vi "GraphXYto2DArrayIndexes.vi"(8 "error in (no error)":errorcluster, 10 "XY":cluster{"X":dbl, "Y":dbl}, 11 "IntensityGraph in":refnum<vi>) -> (0 "error out":errorcluster, 1 "Y Index":i32, 2 "X Index":i32, 3 "reference out":refnum<vi>)   [LabVIEW 2023]
doc: "This VI translates axis position Coord on the graph to it's nearest X and Y pixel index."
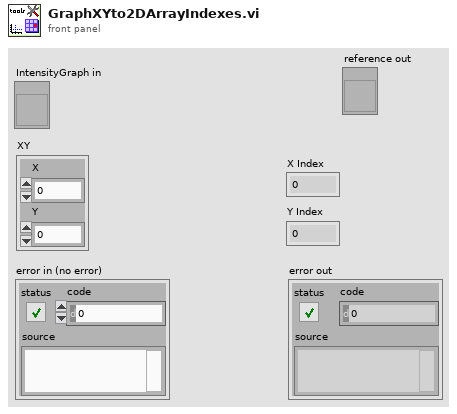
[diagram p1: front panel]
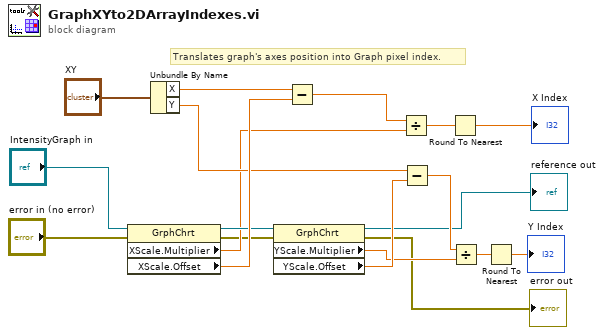
[diagram p0: block diagram]
diagram:
  # "Translates graph's axes position into Graph pixel index."
  n1 = property on="Property Node" class="GrphChrt"(reference="IntensityGraph in", error in="error in (no error)") -> (reference out=w10:refnum<vi>, error out=w4:errorcluster, "XScale.Multiplier"=w8:dbl, "XScale.Offset"=w15:dbl)
  n2 = Unbundle By Name("XY") -> ("X"=w14:dbl, "Y"=w12:dbl)
  n3 = property on="Property Node" class="GrphChrt"(reference=w10, error in=w4) -> (reference out=→"reference out":refnum<vi>, error out=→"error out":errorcluster, "YScale.Multiplier"=w11:dbl, "YScale.Offset"=w13:dbl)
  n4 = Subtract(x=w14, y=w15) -> (x-y=w7:dbl)
  n5 = Divide(x=w7, y=w8) -> (x/y=w16:dbl)
  n6 = Subtract(x=w12, y=w13) -> (x-y=w9:dbl)
  n7 = Round To Nearest(number=w16) -> (nearest integer value=→"X Index":dbl)
  n8 = Divide(x=w9, y=w11) -> (x/y=w17:dbl)
  n9 = Round To Nearest(number=w17) -> (nearest integer value=→"Y Index":dbl)
